vi "Read Cycle_.vi"(8 "error in (no error)":errorcluster, 11 "Update Filter Cycle Params MSG in":refnum<class "Update Filter Cycle Params MSG.lvclass">) -> (0 "error out":errorcluster, 2 "Cycle?":bool, 3 "Update Filter Cycle Params MSG out":refnum<class "Update Filter Cycle Params MSG.lvclass">)   [LabVIEW 2014, in "Controller.lvlib" / "Update Filter Cycle Params MSG.lvclass"]
uses:
  Update Filter Cycle Params MSG.lvclass
  Update Filter Cycle Params MSG.lvclass/Update Filter Cycle Params MSG.ctl
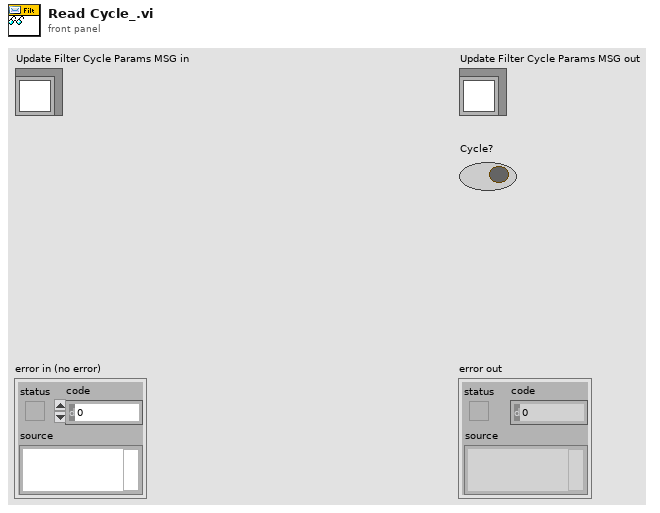
[diagram p1: front panel]
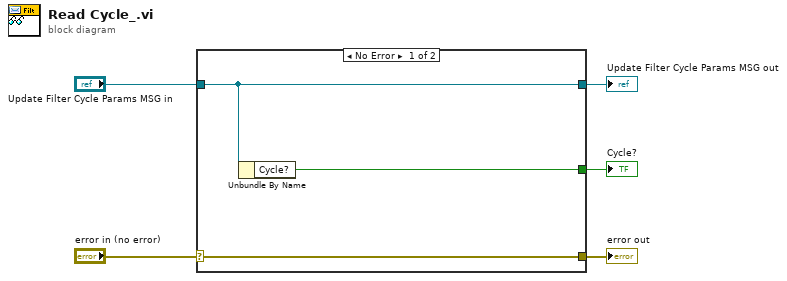
[diagram p0: block diagram]
diagram:
  n1 = case shown="No Error" "error in (no error)" {
    selector: "error in (no error)" -> [w8 w9]
    tunnel: [w8 w9] -> w4
    tunnel: [w7 w10] -> w2
    tunnel: "Update Filter Cycle Params MSG in" -> [w7 w10]
    tunnel: [w6 _] -> w1
    frame No Error {
      n2 = Unbundle By Name(w7) -> ("Cycle?"=w6:bool)
    }
    frame Error {
    }
  }
  "error out" <- w4
  "Update Filter Cycle Params MSG out" <- w2
  "Cycle?" <- w1
